vi "Prompt for Step--UI Interlocks.vi"(8 "error in (no error)":errorcluster, 10 "Control Ref Map":map{string, refnum<vi>}(c390), 11 "Keyboard Action in":refnum<class "Keyboard Action.lvclass">) -> (0 "error out":errorcluster, 2 "Step Valid?":bool, 3 "Keyboard Action out":refnum<class "Keyboard Action.lvclass">)   [LabVIEW 2020, in "MacroAssert.lvlib" / "Keyboard Action.lvclass"]
doc: "Enables or disables buttons within the \"Prompt for Step\" VI according to the current state of the system."
uses:
  Keyboard Action.lvclass
  Support/Get Control Reference by Label (1D STR).vi
  MacroAssert.lvlib
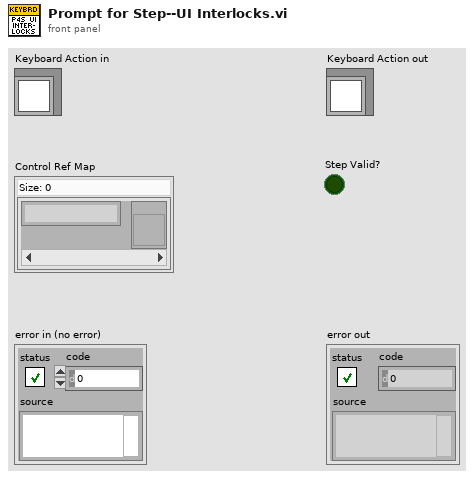
[diagram p1: front panel]
types:
  T1 = typedef "MacroAssert.lvlib/Keyboard Action.lvclass/Keyboard Action Type.ctl" = enum16{"Key Press", "Key Down", "Key Up"}
  T2 = enum8{"Enabled", "Disabled", "Disabled and Grayed Out"}
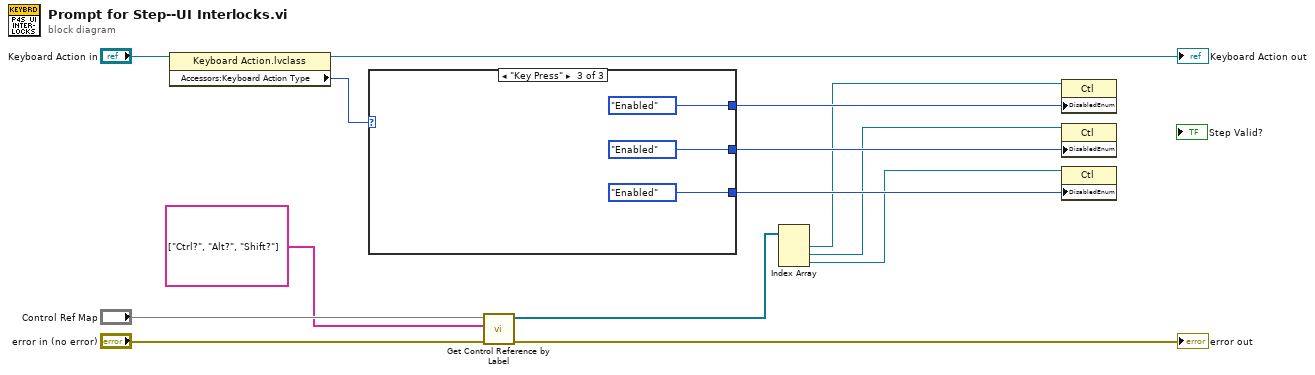
[diagram p0: block diagram]
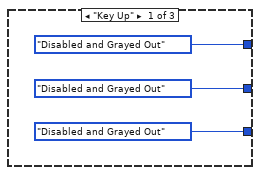
[diagram p2: hidden frame]
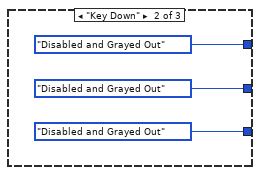
[diagram p3: hidden frame]
diagram:
  n1 = property on="Property Node" class="Keyboard Action.lvclass"(reference="Keyboard Action in") -> (reference out=→"Keyboard Action out":refnum<class "Keyboard Action.lvclass">, "Accessors:Keyboard Action Type"=w12:T1)  [unwired: 1 in, 1 out]
  n2 = case shown="\"Key Press\"" w12 {
    tunnel: [T2."Disabled and Grayed Out" ("Disabled") T2."Disabled and Grayed Out" ("Disabled") T2."Enabled" ("Disabled")] -> w10
    tunnel: [T2."Disabled and Grayed Out" ("Disabled") T2."Disabled and Grayed Out" ("Disabled") T2."Enabled" ("Disabled")] -> w9
    tunnel: [T2."Disabled and Grayed Out" ("Disabled") T2."Disabled and Grayed Out" ("Disabled") T2."Enabled" ("Disabled")] -> w8
    frame "Key Up" {
    }
    frame "Key Down" {
    }
    frame "Key Press" {
    }
  }
  n3 = call-poly "Get Control Reference by Label.vi"("error in (no error)"="error in (no error)", "Control Names"=string[] ["Ctrl?", "Alt?", "Shift?"], "Control Ref Map"="Control Ref Map") -> ("error out"=→"error out":errorcluster, "Control Refs"=w5:refnum<vi>[])  [unwired: 6 in, 1 out]
  n4 = Index Array(array=w5) -> (element #1=w4:refnum<vi>, element #2=w3:refnum<vi>, element #3=w2:refnum<vi>)  [unwired: 3 in]
  n5 = property on="Property Node" class="Ctl"(reference=w4, "DisabledEnum"=w8) -> ()  [unwired: 1 in, 2 out]
  n6 = property on="Property Node" class="Ctl"(reference=w3, "DisabledEnum"=w9) -> ()  [unwired: 1 in, 2 out]
  n7 = property on="Property Node" class="Ctl"(reference=w2, "DisabledEnum"=w10) -> ()  [unwired: 1 in, 2 out]
